vi "Send Generic Message.vi"(8 "error in (no error)":errorcluster, 9 "Message Data":string, 10 "Message Name":string, 11 "Plugin Session in":refnum<class "Plugin Session.lvclass">) -> (0 "error out":errorcluster, 3 "Plugin Session out":refnum<class "Plugin Session.lvclass">)   [LabVIEW 2020, in "InstrumentStudio Plugin SDK.lvlib" / "Plugin Session.lvclass"]
uses:
  Plugin Session.lvclass
  Plugin Session.lvclass/Plugin Session.ctl
  Read Session Id.vi
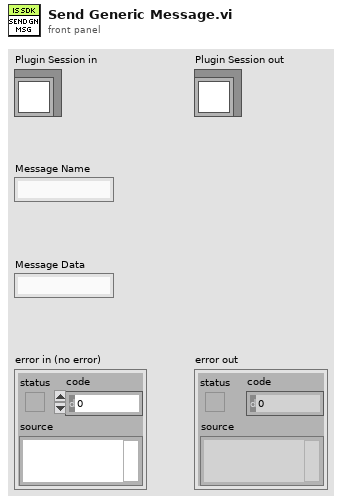
[diagram p1: front panel]
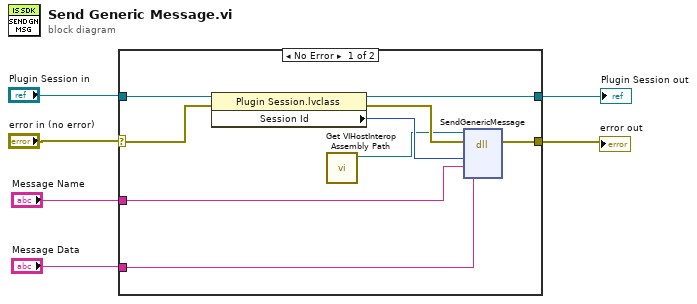
[diagram p0: block diagram]
diagram:
  n1 = case shown="No Error" "error in (no error)" {
    selector: "error in (no error)" -> [w13 w16]
    tunnel: "Plugin Session in" -> [w15 w17]
    tunnel: [w14 w17] -> w4
    tunnel: [w10 w16] -> w3
    tunnel: "Message Name" -> [w9 _]
    tunnel: "Message Data" -> [w8 _]
    frame No Error {
      n2 = property class="Plugin Session.lvclass"(reference=w15, error in=w13) -> (reference out=w14:refnum<class "Plugin Session.lvclass">, error out=w12:errorcluster, "Session Id"=w11:u64)
      n3 = call "Get VIHostInterop Assembly Path.vi"() -> ("VIHost.Interop Assembly"=w7:path)  [unwired: 11 in]
      n4 = dll-call lib="C:/Dev/ASW/Source/InstrumentStudio/IFDistribution/VIHostPanel/objects/export/targets/win64U/x64/msvc-14.0/debug/NationalInstruments.VIHost.Interop.dll" fn="SendGenericMessage"(path in=w7, error in=w12, "sessionId"=w11, "messageName"=w9, "messageData"=w8) -> (error out=w10:errorcluster)  [unwired: 5 in, 1 out]
    }
    frame Error {
    }
  }
  "Plugin Session out" <- w4
  "error out" <- w3
